vi "mav_connection_open.vi"(8 "error in":errorcluster, 9 "Connection Type":enum32{"TCP", "SERIAL", "UDP"}(tab), 11 "mav_connection_in":T2={"serial"={"baudrate"=115200, "visa in"=""}, "tcp"={"address"="127.0.0.1", "port"=5760}, "udp"={"address"="127.0.0.1", "port"=5760}}) -> (0 "error out":errorcluster, 3 "mav_connection_out":T1)   [LabVIEW 2023]
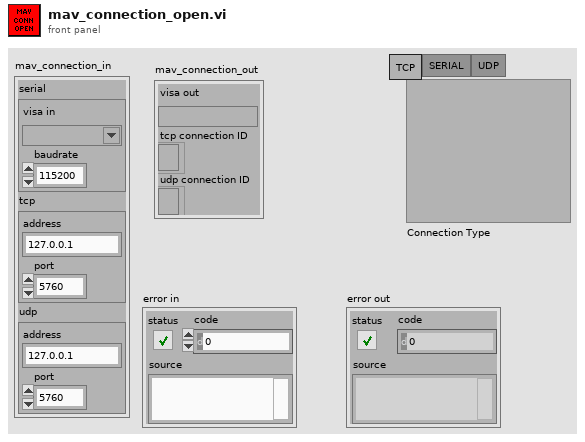
[diagram p1: front panel]
types:
  T1 = cluster{"visa out":refnum<visa-resource-name>, "tcp connection ID":refnum<k5>, "udp connection ID":refnum<k16>}
  T2 = cluster{"serial":cluster{"baudrate":u32, "visa in":refnum<visa-resource-name>}, "tcp":cluster{"address":string, "port":u16}, "udp":cluster{"address":string, "port":u16}}
  T3 = cluster{"baudrate":u32, "visa in":refnum<visa-resource-name>}
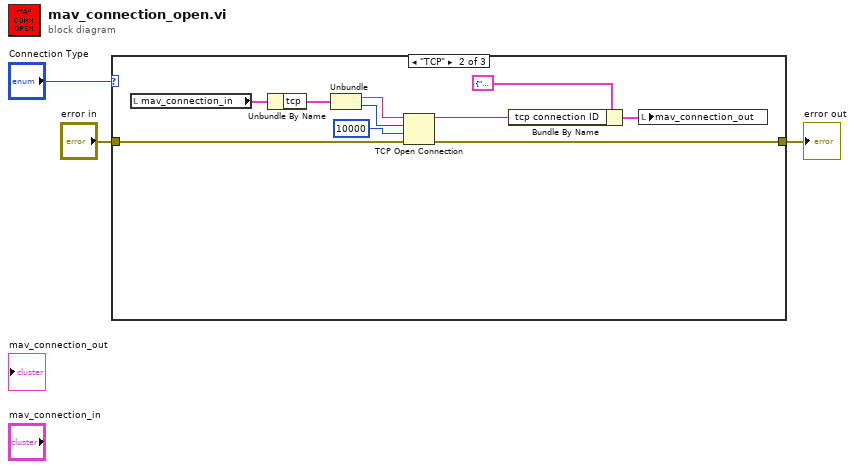
[diagram p0: block diagram]
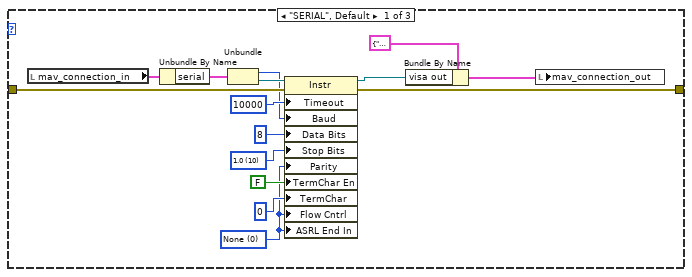
[diagram p2: hidden frame]
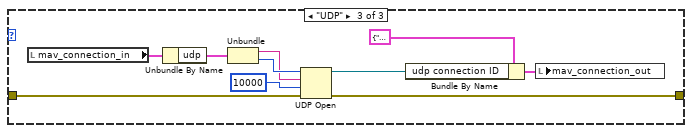
[diagram p3: hidden frame]
diagram:
  n1 = case shown="\"TCP\"" "Connection Type" {
    tunnel: "error in" -> [w12 w24 w30]
    tunnel: [w11 w27 w29] -> w2
    frame "SERIAL", Default {
      w13 = u16 0 items=["None", "Last Bit", "TermChar"] ("Serial Settings:End Mode for Reads")
      w16 = u16 10 items=["1.0"=10, "1.5"=15, "2.0"=20] ("Serial Settings:Stop Bits")
      n2 = local read "mav_connection_in"() -> (w10:T2)
      n3 = Unbundle By Name(w10) -> ("serial"=w9:T3)
      n4 = Unbundle(w9) -> ("baudrate"=w5:u32, "visa in"=w6:refnum<visa-resource-name>)
      n5 = property class="Instr"(reference=w6, error in=w12, "Timeout"=u32 10000 ("General Settings:Timeout Value"), "Baud"=w5, "Data Bits"=u16 8 ("Serial Settings:Data Bits"), "Stop Bits"=w16, "Parity"=w13, "TermChar En"=FALSE ("Message Based Settings:Termination Character Enable"), "TermChar"=u8 0 ("Message Based Settings:Termination Character"), "Flow Cntrl"=w13, "ASRL End In"=w13) -> (reference out=w7:refnum<visa-resource-name>, error out=w11:errorcluster)
      n6 = Bundle By Name(cluster=T1 {"visa out"="", "tcp connection ID"=refnum, "udp connection ID"=refnum} ("mav_connection_out"), "visa out"=w7) -> (w8:T1)
      n7 = local write "mav_connection_out"(w8) -> ()
    }
    frame "TCP" {
      n8 = local read "mav_connection_in"() -> (w23:T2)
      n9 = Unbundle By Name(w23) -> ("tcp"=w22:cluster{"address":string, "port":u16})
      n10 = Unbundle(w22) -> ("address"=w26:string, "port"=w25:u16)
      n11 = TCP Open Connection(address=w26, remote port or service name=w25, timeout ms (60000)=10000, error in (no error)=w24) -> (connection ID=w21:refnum<k5>, error out=w27:errorcluster)  [unwired: 1 in]
      n12 = Bundle By Name(cluster=T1 {"visa out"="", "tcp connection ID"=refnum, "udp connection ID"=refnum} ("mav_connection_out"), "tcp connection ID"=w21) -> (w20:T1)
      n13 = local write "mav_connection_out"(w20) -> ()
    }
    frame "UDP" {
      n14 = local read "mav_connection_in"() -> (w33:T2)
      n15 = Unbundle By Name(w33) -> ("udp"=w34:cluster{"address":string, "port":u16})
      n16 = Unbundle(w34) -> ("address"=w35:string, "port"=w36:u16)
      n17 = UDP Open(8:w30, 9:10000 ("timeout ms (25000)"), 10:w35, 11:w36) -> (port=w37:refnum<k16>, 0:w29:errorcluster)  [unwired: 1 in, 1 out]
      n18 = Bundle By Name(cluster=T1 {"visa out"="", "tcp connection ID"=refnum, "udp connection ID"=refnum} ("mav_connection_out"), "udp connection ID"=w37) -> (w38:T1)
      n19 = local write "mav_connection_out"(w38) -> ()
    }
  }
  "error out" <- w2
